vi "FromIPtoVISA.vi"(3 "VISA in":refnum<visa-resource-name>, 4 "IP input":string="192.168.129.96", 5 "IP to VISA?":bool) -> (0 "IP  out":string="192.168.129.96", 1 "VISA out":refnum<visa-resource-name>)   [LabVIEW 2018]
uses:
  <vilib>/regexp/Match Regular Expression.xnode
panel:
  out "General Settings:Resource Name":string
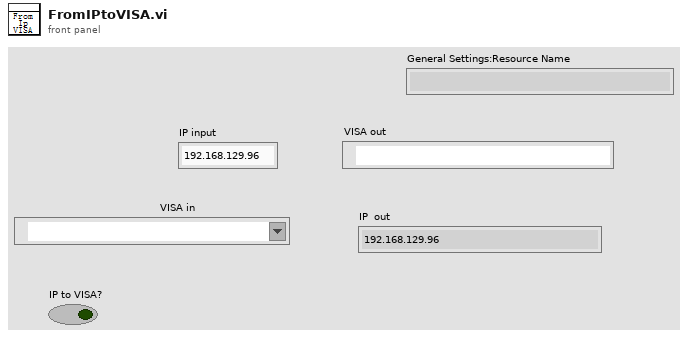
[diagram p1: front panel]
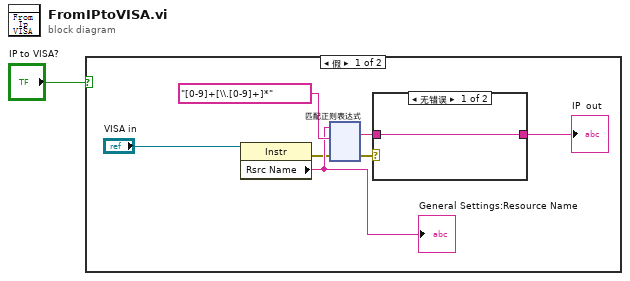
[diagram p0: block diagram]
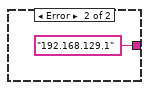
[diagram p2: hidden frame]
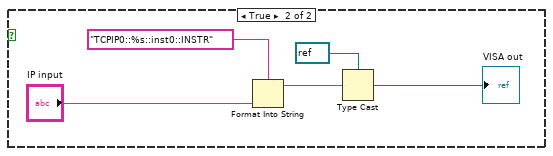
[diagram p3: hidden frame]
diagram:
  n1 = case shown="假" "IP to VISA?" {
    frame False {
      n2 = property class="Instr"(reference="VISA in") -> (error out=w5:errorcluster, "Rsrc Name"=w6:string)  [unwired: 1 in, 1 out]
      "General Settings:Resource Name" <- w6
      n3 = xnode "匹配正则表达式"("输入字符串"=w6, "正则表达式"="[0-9]+[\\.[0-9]+]*" ("Interface Information:Interface Description"), "错误输入"=w5) -> ("所有匹配"=w3:string, "错误输出"=w4:errorcluster)  [unwired: 3 in, 3 out]
      n4 = case shown="无错误" w4 {
        tunnel: w3 -> [w9 _]
        tunnel: [w9 "192.168.129.1" ("所有匹配")] -> w2
        frame No Error {
        }
        frame Error {
        }
      }
      "IP  out" <- w2
    }
    frame True {
      n5 = Format Into String(format string="TCPIP0::%s::inst0::INSTR" ("Interface Information:Interface Description"), "IP input") -> (resulting string=w127:string)  [unwired: 2 in, 1 out]
      n6 = Type Cast(type=refnum<visa-resource-name> refnum ("示波器. 示波器VISA"), x=w127) -> (*(type *) &x=→"VISA out":refnum<visa-resource-name>)
    }
  }
